vi "Output String.vi"(8 "error in (no error)":errorcluster, 9 "position":cluster{"row":i8, "column":i8}, 10 "text":string, 11 "HD44780 in":refnum<class "HD44780.lvclass">) -> (0 "error out":errorcluster, 1 "current cursor position":cluster{"row":i8, "column":i8}, 3 "HD44780 out":refnum<class "HD44780.lvclass">)   [LabVIEW 2017, in "HD44780.lvclass"]
uses:
  HD44780.lvclass
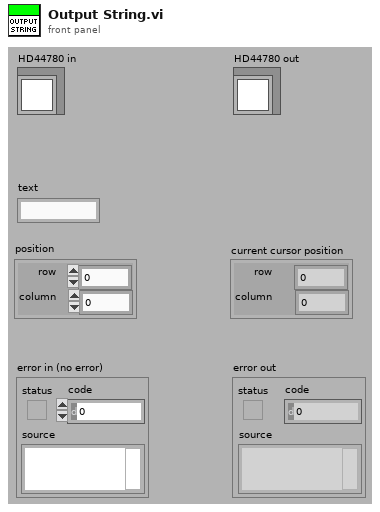
[diagram p1: front panel]
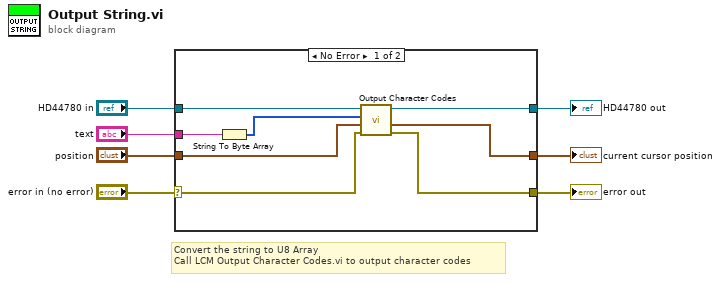
[diagram p0: block diagram]
diagram:
  # "Convert the string to U8 Array\nCall LCM Output Character Codes.vi to output character codes"
  n1 = case shown="No Error" "error in (no error)" {
    selector: "error in (no error)" -> [w10 w18]
    tunnel: [w9 w18] -> w6
    tunnel: [w14 w17] -> w4
    tunnel: "HD44780 in" -> [w15 w17]
    tunnel: "text" -> [w12 _]
    tunnel: "position" -> [w11 w16]
    tunnel: [w8 w16] -> w1
    frame No Error {
      n2 = String To Byte Array(string=w12) -> (unsigned byte array=w13:u8[])
      n3 = call-dynamic "Output Character Codes.vi"("error in (no error)"=w10, "position"=w11, "character codes"=w13, "HD44780 in"=w15) -> ("error out"=w9:errorcluster, "current cursor position"=w8:cluster{"row":i8, "column":i8}, "HD44780 out"=w14:refnum<class "HD44780.lvclass">)  [unwired: 5 in]
    }
    frame Error {
    }
  }
  "error out" <- w6
  "HD44780 out" <- w4
  "current cursor position" <- w1
